vi "Data_get.vi"() -> ()   [LabVIEW 2009]
uses:
  <vilib>/Analysis/2dsp.llb/Real FFT.vi
  <vilib>/Analysis/NI_AALPro.lvlib
panel:
  in  "Chirp up to (GHz)":dbl
  in  "PauseB":bool caption="Pause"
  in  "Substr":bool
  out "tdsavges#":i32 caption="tds averaged:"
  in  "Auto":bool caption="Autosave"
  in  "FFT every#":u32=1 min=1 max=1000 step=1
  in  "#steps":u32=1 min=1 step=1
  in  "f step (MHz)":dbl=0.0003 min=0.00025 max=67.0 step=1e-06 format="%#.12f"
  in  "ps/point":T1(ring)
  in  "ns/div":T2(ring)
  out "Current sweep":u32=1 min=1 max=1000 step=1
  in  "Ext":string="ccd"
  out "f cur. (MHz)":string
  in  "Name":string="trace"
  in  "Folder":path
  in  "#Sweeps":u32=1 min=1 max=1000 step=1
  in  "Ampl. (dBm)":dbl min=-135.0 max=30.0 step=0.5 format="%#_8g"
  in  "f start (MHz)":dbl=0.0003 min=0.00025 max=67.0 step=1e-06 format="%#.12f"
  in  "Start":bool
  in  "Quit":bool
  in  "E8257D VISA Port":refnum<visa-resource-name>="GPIB0::1::INSTR"
  out "read time (ms)":u32
  out "#points":u32
  out "Busy":bool
  in  "Repetition rate (Hz)":ext=2.5
  in  "Chirp start (MHz)":ext=2.5
  in  "Filter up to (MHz)":ext=2.5
  in  "Amount of averagings":u32=10 min=1 step=1
  out "Data":dbl[](array[numeric])
  out "XY Graph 5":cluster{ext[], dbl[]}(graph)
  out "FFT (Im)":dbl[](array[numeric])
  out "FFT (Re)":dbl[](array[numeric])
  out "Final array":ext[][](array[numeric])
  out "size(s)":i32
  out "Oscilloscope Data":dbl[](array[numeric])
  in  "Channel Number":u16=1
  out "Oscilloscope graph":dbl[](graph)
  in  "Stop":bool
  in  "TDS VISA Port":refnum<visa-resource-name>="GPIB0::1::INSTR"
  # "TDS6000"
  # "E8257D"
  # "File Storage"
  # "Control"
  # "Spectrum data"
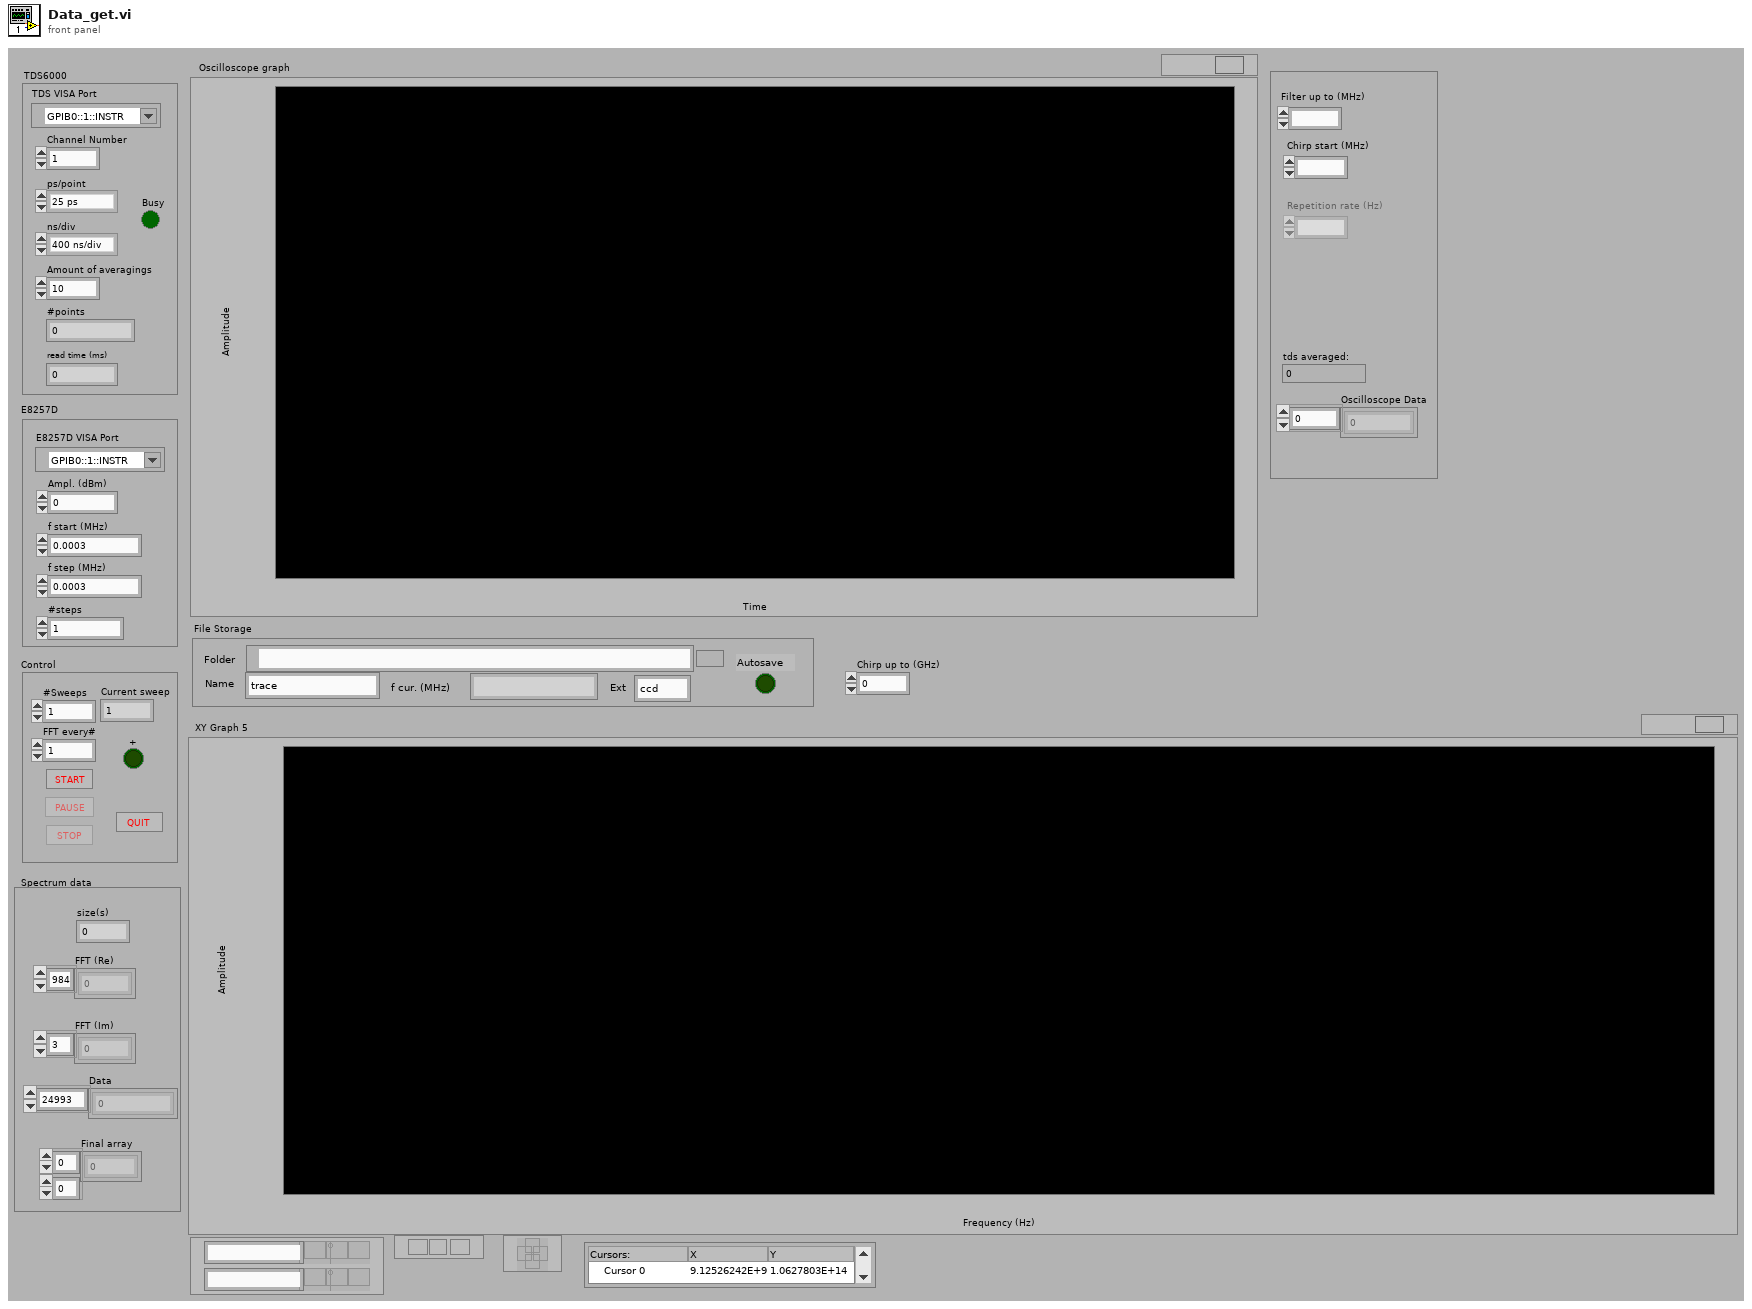
[diagram p1: front panel]
types:
  T1 = enum16{"25 ps", "50 ps", "100 ps", "200 ps", "400 ps", "800 ps", "2 ns"}
  T2 = enum16{"400 ns/div", "1 us/div", "2 us/div", "4 us/div", "10 us/div", "20 us/div"}
  T3 = enum8{"Enabled", "Disabled", "Disabled and Grayed Out"}
  T4 = enum16{"open", "replace", "create", "open or create", "replace or create", "replace or create with confirmation"}
  T5 = cluster{"Folder":path, "Name":string, "Ext":string}
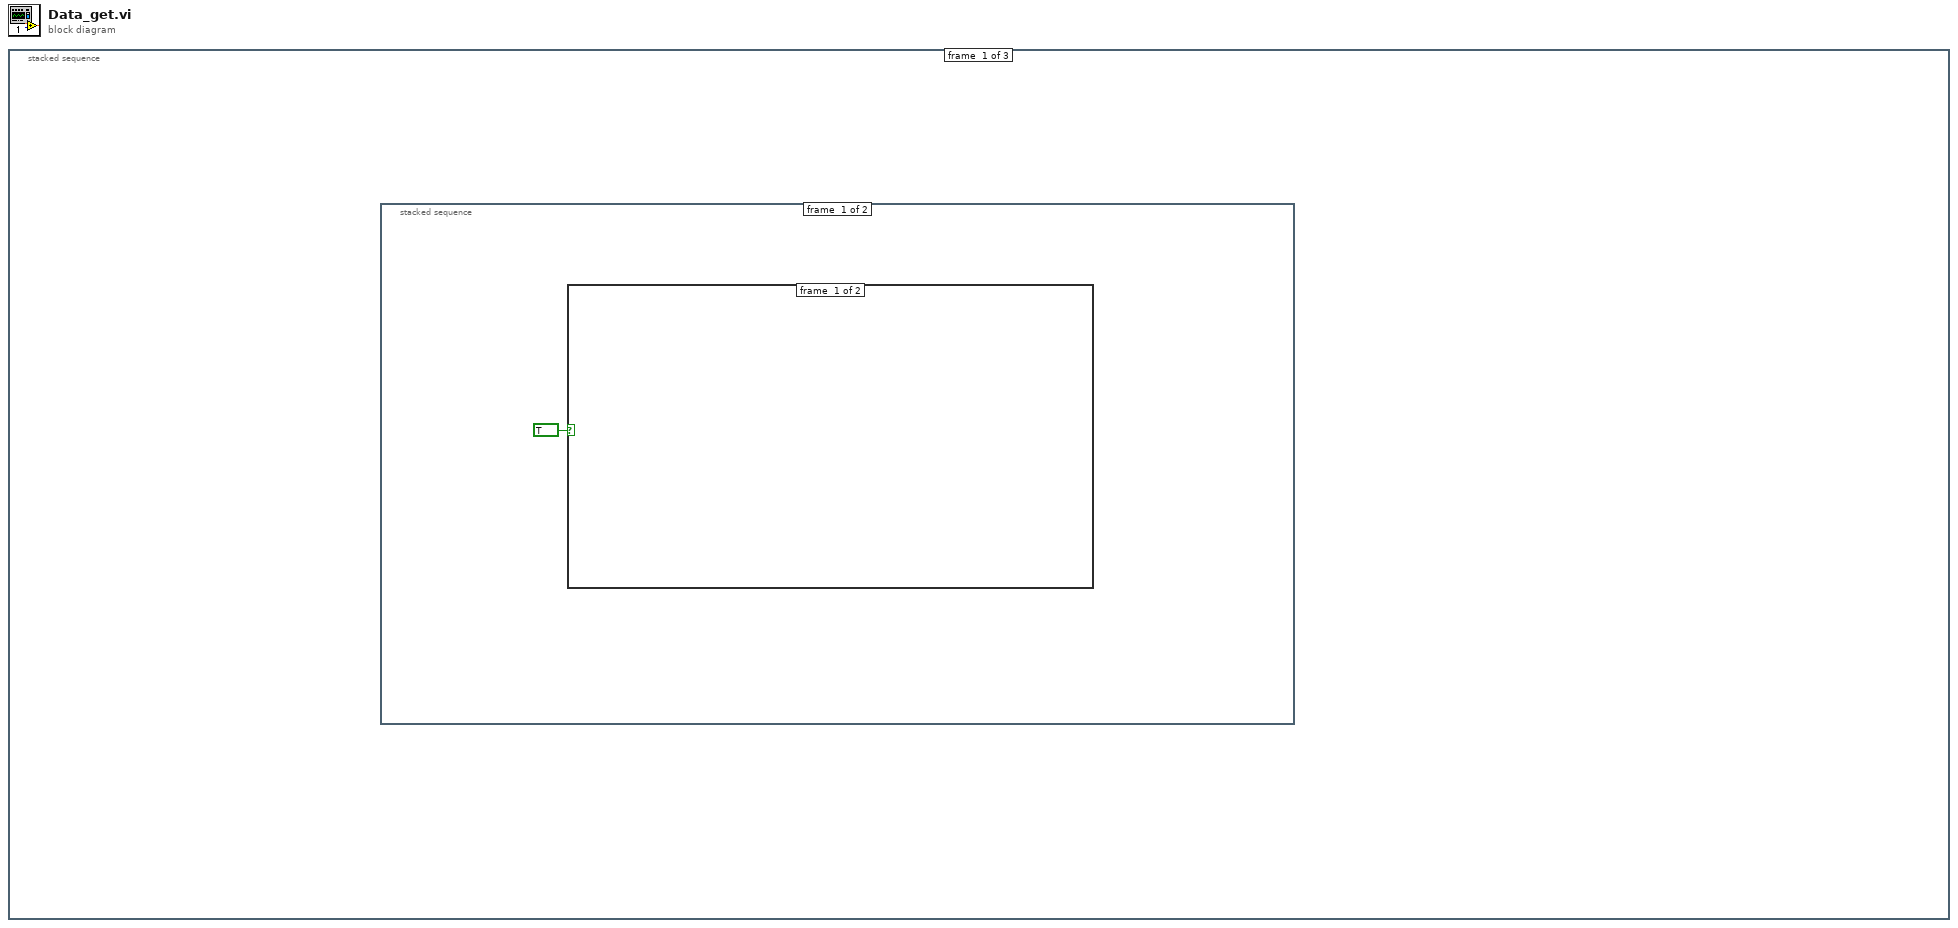
[diagram p0: block diagram]
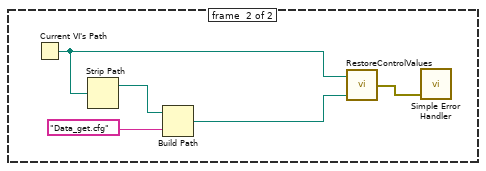
[diagram p2: hidden frame]
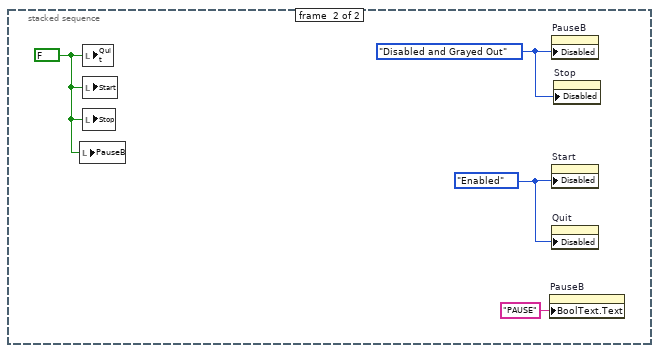
[diagram p3: hidden frame]
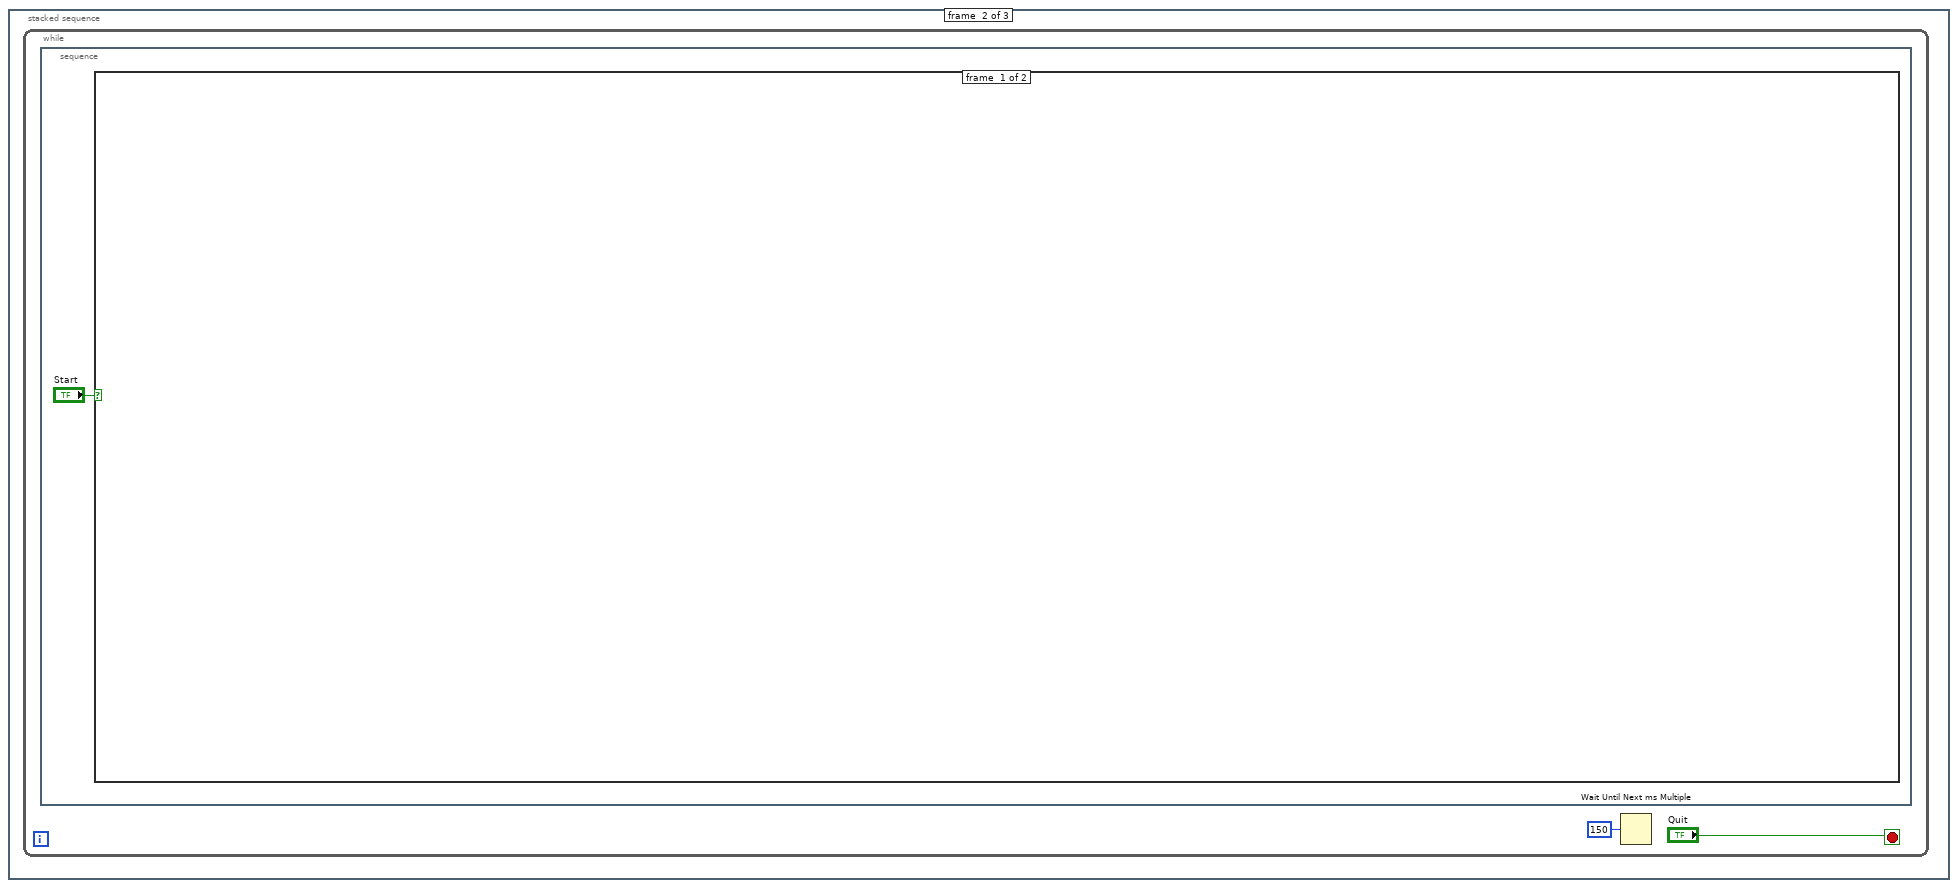
[diagram p4: hidden frame]
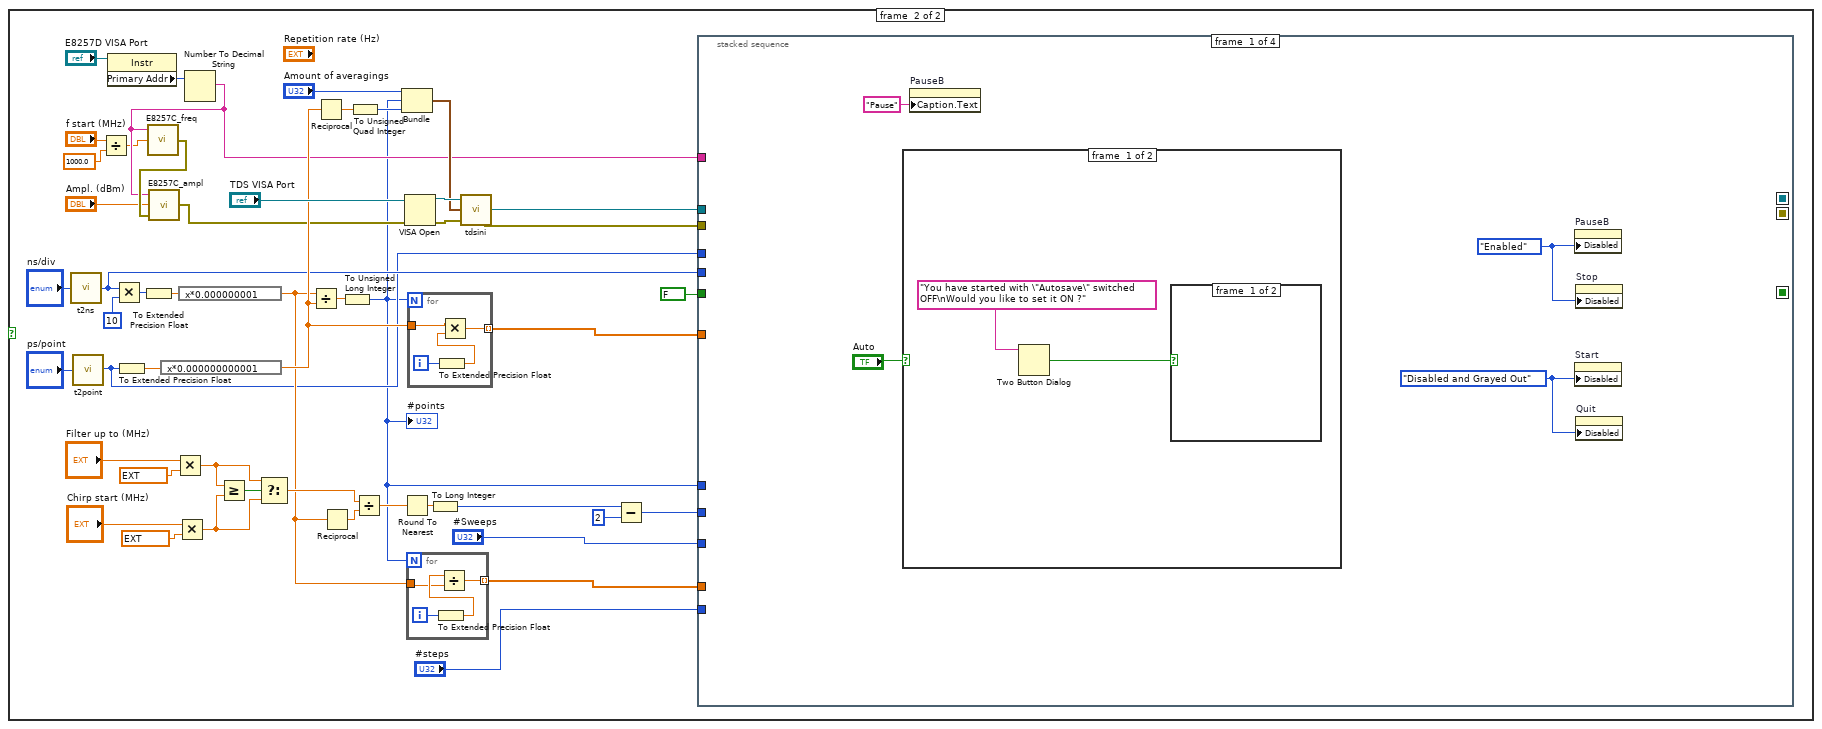
[diagram p5: hidden frame]
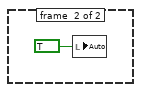
[diagram p6: hidden frame]
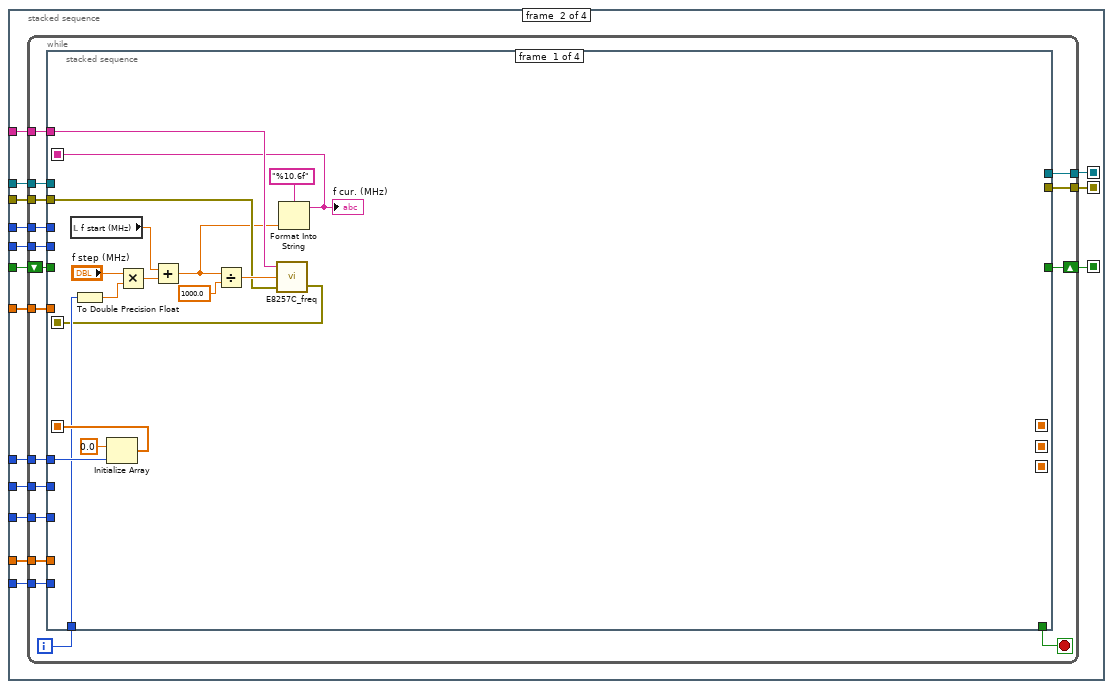
[diagram p8: hidden frame]
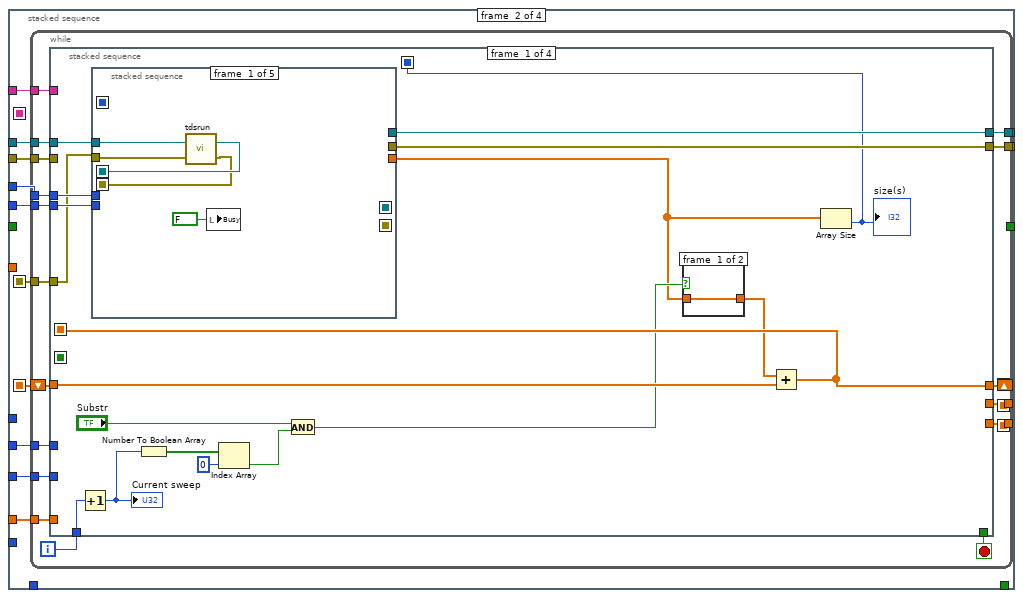
[diagram p9: hidden frame]
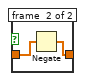
[diagram p10: hidden frame]
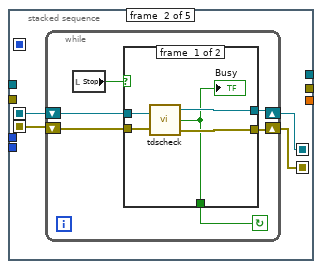
[diagram p11: hidden frame]
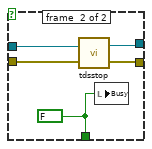
[diagram p12: hidden frame]
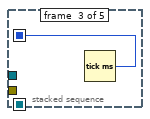
[diagram p13: hidden frame]
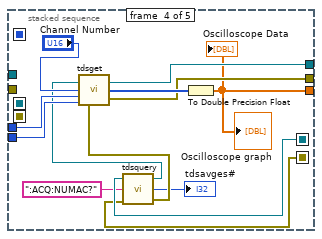
[diagram p14: hidden frame]
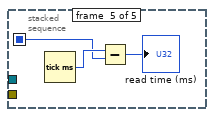
[diagram p15: hidden frame]
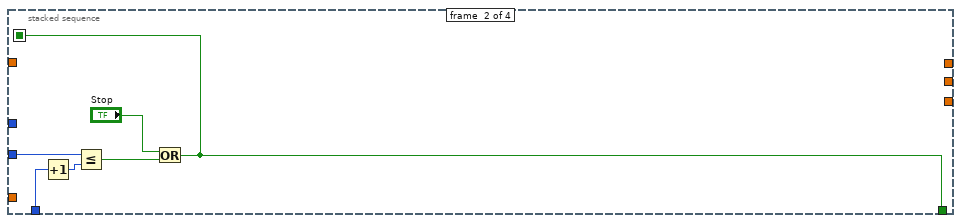
[diagram p16: hidden frame]
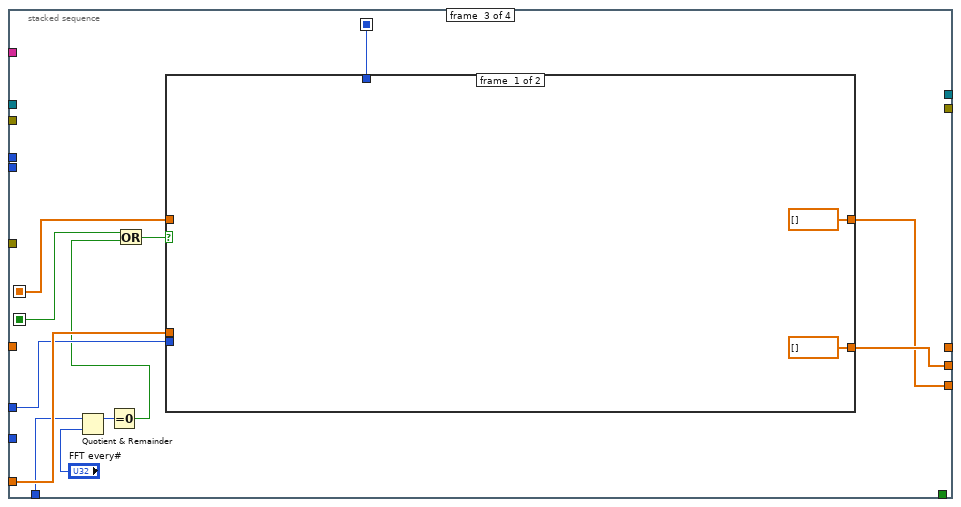
[diagram p17: hidden frame]
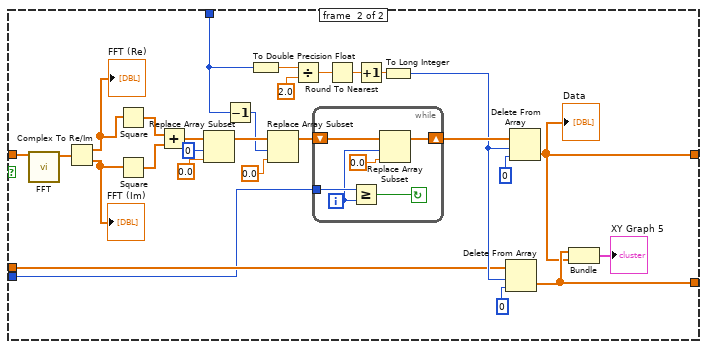
[diagram p18: hidden frame]
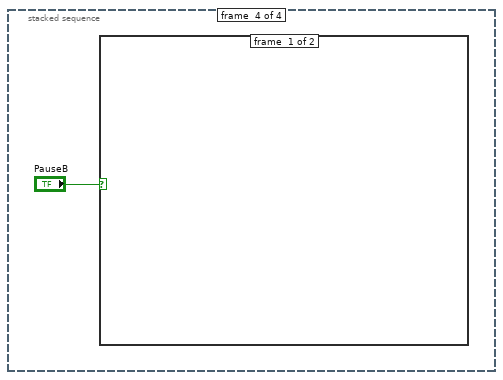
[diagram p19: hidden frame]
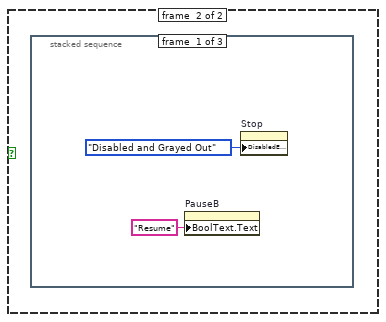
[diagram p20: hidden frame]
diagram:
  n1 = stacked-sequence {
    frame #0 {
      n2 = stacked-sequence {
        frame #0 {
          n3 = case shown="True" TRUE {
            frame #0 {
            }
            frame #1 {
              n4 = Current VI's Path() -> (path=w2:path)
              n5 = Strip Path(path=w2) -> (stripped path=w3:path)  [unwired: 1 out]
              n6 = Build Path(base path=w3, name or relative path="Data_get.cfg") -> (appended path=w5:path)
              n7 = call "RestoreControlValues.vi"("file path"=w5, "vi path"=w2) -> ("error out"=w4:errorcluster)
              n8 = call <vilib>:"Simple Error Handler.vi"("error in (no error)"=w4) -> ()  [unwired: 4 in, 5 out]
            }
          }
        }
        frame #1 {
          w9 = T3."Disabled and Grayed Out" ("Disabled")
          w7 = T3."Enabled" ("Disabled")
          w10 = FALSE ("Quit")
          n9 = local write "PauseB"(w10) -> ()
          n10 = local write "Quit"(w10) -> ()
          n11 = local write "Start"(w10) -> ()
          n12 = local write "Stop"(w10) -> ()
          n13 = property on="PauseB" class="Bool (strict)"("BoolText.Text"="PAUSE" ("Boolean Text.Text")) -> ()  [unwired: 2 in, 2 out]
          n14 = property on="PauseB" class="Bool (strict)"("Disabled"=w9) -> ()  [unwired: 2 in, 2 out]
          n15 = property on="Start" class="Bool (strict)"("Disabled"=w7) -> ()  [unwired: 2 in, 2 out]
          n16 = property on="Quit" class="Bool (strict)"("Disabled"=w7) -> ()  [unwired: 2 in, 2 out]
          n17 = property on="Stop" class="Bool (strict)"("Disabled"=w9) -> ()  [unwired: 2 in, 2 out]
        }
      }
    }
    frame #1 {
      n18 = while {
        stop <- "Quit" stop-if-true
        n19 = stacked-sequence {
          frame #0 {
            n20 = case shown="True" "Start" {
              frame #0 {
              }
              frame #1 {
                n21 = call "t2ns.vi"("t/div"="ns/div") -> ("ns/div"=w23:u32)
                n22 = call "t2point.vi"("t/point"="ps/point") -> ("ps/point"=w21:u32)
                n23 = Divide(x="f start (MHz)", y=1000.0) -> (x/y=w26:dbl)
                n24 = property class="Instr"(reference="E8257D VISA Port") -> ("Primary Addr"=w33:u16)  [unwired: 1 in, 2 out]
                n25 = Multiply(x=w23, y=u32 10) -> (x*y=w56:u32)
                n26 = To Extended Precision Float(1:w21) -> (0:w53:ext)
                n27 = To Extended Precision Float(1:w56) -> (0:w54:ext)
                n28 = expression code="x*0.000000000001"(w53) -> (w39:ext)
                n29 = Multiply(x="Filter up to (MHz)", y=ext 1000000.0) -> (x*y=w45:ext)
                n30 = Multiply(x="Chirp start (MHz)", y=ext 1000000.0) -> (x*y=w42:ext)
                n31 = expression code="x*0.000000001"(w54) -> (w35:ext)
                n32 = Number To Decimal String(number=w33) -> (decimal integer string=w30:string)  [unwired: 1 in]
                n33 = call "E8257C_freq.vi"("Frequency GHz"=w26, "GPIB address"=w30) -> ("error out"=w31:errorcluster)  [unwired: 1 in]
                n34 = call "E8257C_ampl.vi"("error in"=w31, "Amplitude dBm"="Ampl. (dBm)", "GPIB address"=w30) -> ("error out"=w29:errorcluster)
                n35 = Greater Or Equal?(x=w45, y=w42) -> (x >= y?=w52:bool)
                n36 = Select(t=w45, s=w52, f=w42) -> (s? t:f=w50:ext)
                n37 = Divide(x=w35, y=w39) -> (x/y=w55:ext)
                n38 = Reciprocal(x=w39) -> (1/x=w37:ext)
                n39 = Reciprocal(x=w35) -> (1/x=w51:ext)
                n40 = To Unsigned Long Integer(number=w55) -> (unsigned 32bit integer=w19:u32)
                "#points" <- w19
                n41 = To Unsigned Quad Integer(1:w37) -> (0:w38:u64)
                n42 = Divide(x=w50, y=w51) -> (x/y=w49:ext)
                n43 = Bundle("Amount of averagings"="Amount of averagings", w19, w38) -> (w40:cluster{"Amount of averagings ":u32, u32, u64})  [unwired: 1 in]
                n44 = Round To Nearest(number=w49) -> (nearest integer value=w48:ext)
                n45 = VISA Open(error in (no error)=w29, VISA resource name="TDS VISA Port") -> (VISA resource name=w59:refnum<visa-resource-name>, error out=w60:errorcluster)  [unwired: 3 in]
                n46 = for {
                  N: w19 -> [_]
                  tunnel: w35 -> [w468]
                  tunnel: [w470] -> w36 mode=indexing
                  i -> [w471]
                  n47 = To Extended Precision Float(1:w471) -> (0:w469:ext)
                  n48 = Divide(x=w469, y=w468) -> (x/y=w470:ext)
                }
                n49 = for {
                  N: w19 -> [_]
                  tunnel: w39 -> [w473]
                  tunnel: [w472] -> w24 mode=indexing
                  i -> [w475]
                  n50 = To Extended Precision Float(1:w475) -> (0:w474:ext)
                  n51 = Multiply(x=w473, y=w474) -> (x*y=w472:ext)
                }
                n52 = To Long Integer(number=w48) -> (32bit integer=w16:i32)
                n53 = call "tdsini.vi"("Error In (No Error)"=w60, "Acq_par"=w40, "VISA Port In"=w59) -> ("Error Out"=w61:errorcluster, "VISA Port Out"=w62:refnum<visa-resource-name>)
                n54 = Subtract(x=w16, y=2) -> (x-y=w14:i32)
                n55 = stacked-sequence {
                  seq-local: [_ w76 _ _] -> [_ _ w429 _]
                  seq-local: [_ w75 _ _] -> [_ _ w428 _]
                  seq-local: [_ w70 _ _] -> [_ _ _ w430]
                  tunnel: w62 -> [_ w84 _ _]
                  tunnel: w61 -> [_ w83 _ _]
                  tunnel: w21 -> [_ w82 _ _]
                  tunnel: w23 -> [_ w81 _ _]
                  tunnel: w14 -> [_ w80 _ _]
                  tunnel: w36 -> [_ w79 _ _]
                  tunnel: w30 -> [_ w78 w426 _]
                  tunnel: "#Sweeps" -> [_ w77 _ _]
                  tunnel: w24 -> [_ w72 _ _]
                  tunnel: w19 -> [_ w74 _ _]
                  tunnel: "#steps" -> [_ w73 _ _]
                  tunnel: FALSE -> [_ w71 _ _]
                  frame #0 {
                    w64 = T3."Enabled" ("Disabled")
                    w63 = T3."Disabled and Grayed Out" ("Disabled")
                    n56 = case shown="False" "Auto" {
                      frame #0 {
                        n57 = Two Button Dialog(message="You have started with \"Autosave\" switched OFF\nWould you like to set it ON ?") -> (T button?=w67:bool)  [unwired: 2 in]
                        n58 = case shown="True" w67 {
                          frame #0 {
                          }
                          frame #1 {
                            n59 = local write "Auto"(TRUE) -> ()
                          }
                        }
                      }
                      frame #1 {
                      }
                    }
                    n60 = property on="PauseB" class="Bool (strict)"("Caption.Text"="Pause") -> ()  [unwired: 2 in, 2 out]
                    n61 = property on="PauseB" class="Bool (strict)"("Disabled"=w64) -> ()  [unwired: 2 in, 2 out]
                    n62 = property on="Start" class="Bool (strict)"("Disabled"=w63) -> ()  [unwired: 2 in, 2 out]
                    n63 = property on="Stop" class="Bool (strict)"("Disabled"=w64) -> ()  [unwired: 2 in, 2 out]
                    n64 = property on="Quit" class="Bool (strict)"("Disabled"=w63) -> ()  [unwired: 2 in, 2 out]
                  }
                  frame #1 {
                    n65 = while {
                      tunnel: w84 -> [w101]
                      tunnel: w83 -> [w100]
                      tunnel: w82 -> [w99]
                      tunnel: w81 -> [w98]
                      tunnel: w80 -> [w97]
                      tunnel: w79 -> [w96]
                      tunnel: w78 -> [w95]
                      tunnel: w77 -> [w94]
                      tunnel: [w93] -> w76
                      tunnel: [w92] -> w75
                      tunnel: w74 -> [w91]
                      tunnel: w73 -> [w89]
                      tunnel: w72 -> [w87]
                      shift-right: [w85] -> w70
                      shift-left: w71 -> [w86]
                      i -> [w90]
                      stop <- w88 stop-if-true
                      n66 = stacked-sequence {
                        seq-local: [w116 _ _ _] -> [_ w122 _ _]
                        seq-local: [w105 _ _ _] -> [_ w121 _ _]
                        seq-local: [_ w120 _ _] -> [_ _ w280 _]
                        seq-local: [_ w119 _ _] -> [_ _ w279 _]
                        seq-local: [_ w118 _ _] -> [_ _ w278 _]
                        seq-local: [w102 _ _ _] -> [_ _ w277 _]
                        tunnel: w101 -> [_ w132 _ _]
                        tunnel: w100 -> [w106 w131 _ _]
                        tunnel: w99 -> [_ w130 _ _]
                        tunnel: w98 -> [_ w129 _ _]
                        tunnel: w97 -> [_ w128 _ _]
                        tunnel: w96 -> [_ w127 _ _]
                        tunnel: w95 -> [w107 w126 _ _]
                        tunnel: w94 -> [_ w125 _ _]
                        tunnel: [_ w124 _ _] -> w93
                        tunnel: [_ w123 _ _] -> w92
                        tunnel: w91 -> [w115 _ _ _]
                        tunnel: w90 -> [w110 _ _ w420]
                        tunnel: w89 -> [_ _ _ w419]
                        tunnel: [_ _ _ w418] -> w88
                        tunnel: w87 -> [_ _ w281 _]
                        tunnel: w86 -> [_ _ w275 _]
                        tunnel: [_ _ w274 _] -> w85
                        frame #0 {
                          n67 = local read "f start (MHz)"() -> (w108:dbl)
                          n68 = To Double Precision Float(number=w110) -> (double precision float=w111:dbl)
                          n69 = Initialize Array(0.0 ("element"), w115) -> (w116:dbl[])
                          n70 = Multiply(x="f step (MHz)", y=w111) -> (x*y=w109:dbl)
                          n71 = Add(x=w108, y=w109) -> (x+y=w104:dbl)
                          n72 = Divide(x=w104, y=1000.0) -> (x/y=w114:dbl)
                          n73 = call "E8257C_freq.vi"("error in"=w106, "Frequency GHz"=w114, "GPIB address"=w107) -> ("error out"=w105:errorcluster)
                          n74 = Format Into String(format string="%10.6f", w104) -> (resulting string=w102:string)  [unwired: 2 in, 1 out]
                          "f cur. (MHz)" <- w102
                        }
                        frame #1 {
                          n75 = while {
                            tunnel: [w146] -> w123
                            tunnel: [w147] -> w124
                            tunnel: w131 -> [w148]
                            tunnel: w132 -> [w149]
                            tunnel: w130 -> [w145]
                            tunnel: w129 -> [w144]
                            tunnel: w127 -> [w142]
                            tunnel: w128 -> [w143]
                            tunnel: w126 -> [w139]
                            tunnel: w125 -> [w138]
                            shift-right: [w136] -> w120
                            shift-left: w122 -> [w137]
                            tunnel: [w135] -> w119
                            tunnel: w121 -> [w134]
                            tunnel: [w133] -> w118
                            i -> [w141]
                            stop <- w140 stop-if-true
                            n76 = stacked-sequence {
                              seq-local: [w159 _ _ _] -> [_ _ w230 _]
                              seq-local: [w160 _ _ _] -> [_ _ w229 _]
                              seq-local: [_ w213 _ _] -> [_ _ w220 _]
                              tunnel: w149 -> [w167 _ _ _]
                              tunnel: w148 -> [_ _ _ _]
                              tunnel: [w166 _ _ _] -> w147
                              tunnel: [w165 _ _ _] -> w146
                              tunnel: w145 -> [w164 _ _ _]
                              tunnel: w144 -> [w163 _ _ _]
                              tunnel: w143 -> [_ _ w227 _]
                              tunnel: w142 -> [_ _ w228 _]
                              tunnel: w141 -> [w158 w218 w224 _]
                              tunnel: [_ w213 _ _] -> w140
                              tunnel: w139 -> [_ _ _ _]
                              tunnel: w138 -> [_ w215 _ _]
                              tunnel: w137 -> [w162 _ _ _]
                              tunnel: [w160 _ _ _] -> w136
                              tunnel: [_ _ w226 _] -> w135
                              tunnel: w134 -> [w161 _ _ _]
                              tunnel: [_ _ w225 _] -> w133
                              frame #0 {
                                n77 = Increment(x=w158) -> (x+1=w150:i32)
                                "Current sweep" <- w150
                                n78 = stacked-sequence {
                                seq-local: [w173 _ _ _ _] -> [_ w179 _ _ _]
                                seq-local: [w172 _ _ _ _] -> [_ w178 _ _ _]
                                seq-local: [_ w176 _ _ _] -> [_ _ _ w201 _]
                                seq-local: [_ w177 _ _ _] -> [_ _ _ w202 _]
                                seq-local: [_ _ w196 _ _] -> [_ _ _ _ w211]
                                tunnel: w167 -> [w174 _ _ _ _]
                                tunnel: w161 -> [w175 _ _ _ _]
                                tunnel: [_ _ _ w208 _] -> w166
                                tunnel: [_ _ _ w207 _] -> w165
                                tunnel: w164 -> [_ _ _ w205 _]
                                tunnel: w163 -> [_ _ _ w204 _]
                                tunnel: [_ _ _ w203 _] -> w153
                                frame #0 {
                                n79 = call "tdsrun.vi"("Error In (No Error)"=w175, "VISA Port In"=w174) -> ("Error Out"=w172:errorcluster, "VISA Port Out"=w173:refnum<visa-resource-name>)
                                n80 = local write "Busy"(FALSE ("Busy")) -> ()
                                }
                                frame #1 {
                                n81 = while {
                                shift-right: [w183] -> w177
                                shift-left: w179 -> [w184]
                                shift-right: [w182] -> w176
                                shift-left: w178 -> [w185]
                                stop <- w181 continue-if-true
                                n82 = local read "Stop"() -> (w180:bool)
                                n83 = case shown="True" w180 {
                                tunnel: w185 -> [w190 w194]
                                tunnel: w184 -> [w189 w195]
                                tunnel: [w188 w192] -> w183
                                tunnel: [w187 w193] -> w182
                                tunnel: [w186 w191] -> w181
                                frame #0 {
                                n84 = call "tdscheck.vi"("VISA Port In"=w189, "Error In (No Error)"=w190) -> ("VISA Port Out"=w188:refnum<visa-resource-name>, "busy"=w186:bool, "Error Out"=w187:errorcluster)
                                "Busy" <- w186
                                }
                                frame #1 {
                                w191 = FALSE ("busy")
                                n85 = call "tdsstop.vi"("Error In (No Error)"=w194, "VISA Port In"=w195) -> ("Error Out"=w193:errorcluster, "VISA Port Out"=w192:refnum<visa-resource-name>)
                                n86 = local write "Busy"(w191) -> ()
                                }
                                }
                                }
                                }
                                frame #2 {
                                n87 = Tick Count (ms)() -> (millisecond timer value=w196:u32)
                                }
                                frame #3 {
                                n88 = call "tdsquery.vi"("Error In (No Error)"=w201, "String to TDS"=":ACQ:NUMAC?", "VISA Port In"=w202) -> ("Error Out"=w198:errorcluster, "number"=→"tdsavges#":i32, "VISA Port Out"=w199:refnum<visa-resource-name>)
                                n89 = call "tdsget.vi"("VISA Port In"=w199, "Channel Number"="Channel Number", "ps/point"=w205, "ns/div"=w204, "Error In (No Error)"=w198) -> ("VISA Port Out"=w208:refnum<visa-resource-name>, "TDS Data"=w209:u16[], "Error Out"=w207:errorcluster)  [unwired: 8 in]
                                n90 = To Double Precision Float(number=w209) -> (double precision float=w203:dbl[])
                                "Oscilloscope graph" <- w203
                                "Oscilloscope Data" <- w203
                                }
                                frame #4 {
                                n91 = Tick Count (ms)() -> (millisecond timer value=w212:u32)
                                n92 = Subtract(x=w212, y=w211) -> (x-y=→"read time (ms)":u32)
                                }
                                }
                                n93 = Number To Boolean Array(number=w150) -> (Boolean array=w157:bool[])
                                n94 = Index Array(array=w157, index=0) -> (element=w155:bool)
                                n95 = And(x="Substr", y=w155) -> (x .and. y?=w154:bool)
                                n96 = case shown="True" w154 {
                                tunnel: w153 -> [w168 w170]
                                tunnel: [w168 w169] -> w152
                                frame #0 {
                                }
                                frame #1 {
                                n97 = Negate(x=w170) -> (-x=w169:dbl[])
                                }
                                }
                                n98 = Add(x=w152, y=w162) -> (x+y=w160:dbl[])
                                n99 = Array Size(array=w153) -> (size(s)=w159:i32)
                                "size(s)" <- w159
                              }
                              frame #1 {
                                n100 = Increment(x=w218) -> (x+1=w214:i32)
                                n101 = Less Or Equal?(x=w215, y=w214) -> (x <= y?=w217:bool)
                                n102 = Or(x="Stop", y=w217) -> (x .or. y?=w213:bool)
                              }
                              frame #2 {
                                n103 = Quotient & Remainder(x=w224, y="FFT every#") -> (x-y*floor(x/y)=w222:u32)  [unwired: 1 out]
                                n104 = Equal To 0?(x=w222) -> (x = 0?=w219:bool)
                                n105 = Or(x=w220, y=w219) -> (x .or. y?=w221:bool)
                                n106 = case shown="True" w221 {
                                tunnel: w230 -> [_ w238]
                                tunnel: w229 -> [_ w237]
                                tunnel: w228 -> [_ w236]
                                tunnel: w227 -> [_ w235]
                                tunnel: [ext[] [] w234] -> w226
                                tunnel: [dbl[] [] w233] -> w225
                                frame #0 {
                                }
                                frame #1 {
                                n107 = call-poly <vilib>:"FFT.vi"("X"=w237) -> ("FFT {X}"=w260:cdb[])  [unwired: 9 in, 1 out]
                                n108 = Complex To Re/Im(x + iy=w260) -> (x=w259:dbl[], y=w258:dbl[])
                                "FFT (Re)" <- w259
                                "FFT (Im)" <- w258
                                n109 = Square(x=w259) -> (x^2=w257:dbl[])
                                n110 = Square(x=w258) -> (x^2=w256:dbl[])
                                n111 = Add(x=w257, y=w256) -> (x+y=w252:dbl[])
                                n112 = Replace Array Subset(array=w252, new element=0.0 ("new element/subarray"), index=0) -> (w251:dbl[])
                                n113 = Decrement(x=w238) -> (x-1=w250:i32)
                                n114 = To Double Precision Float(number=w238) -> (double precision float=w246:dbl)
                                n115 = Replace Array Subset(array=w251, new element=0.0 ("new element/subarray"), index=w250) -> (w248:dbl[])
                                n116 = Divide(x=w246, y=2.0) -> (x/y=w244:dbl)
                                n117 = while {
                                tunnel: w235 -> [w265]
                                shift-right: [w263] -> w247
                                shift-left: w248 -> [w264]
                                i -> [w262]
                                stop <- w266 continue-if-true
                                n118 = Greater Or Equal?(x=w265, y=w262) -> (x >= y?=w266:bool)
                                n119 = Replace Array Subset(array=w264, new element=0.0 ("new element/subarray"), index=w262) -> (w263:dbl[])
                                }
                                n120 = Round To Nearest(number=w244) -> (nearest integer value=w243:dbl)
                                n121 = Increment(x=w243) -> (x+1=w242:dbl)
                                n122 = To Long Integer(number=w242) -> (32bit integer=w239:i32)
                                n123 = Delete From Array(array=w236, length=w239, index=0) -> (deleted portion=w234:ext[])  [unwired: 1 out]
                                n124 = Delete From Array(array=w247, length=w239, index=0) -> (deleted portion=w233:dbl[])  [unwired: 1 out]
                                "Data" <- w233
                                n125 = Bundle(w234, w233) -> (→"XY Graph 5":cluster{ext[], dbl[]})  [unwired: 1 in]
                                }
                                }
                              }
                              frame #3 {
                                n126 = case shown="True" "PauseB" {
                                frame #0 {
                                }
                                frame #1 {
                                n127 = stacked-sequence {
                                frame #0 {
                                n128 = property on="PauseB" class="Bool (strict)"("BoolText.Text"="Resume" ("Caption.Text")) -> ()  [unwired: 2 in, 2 out]
                                n129 = property on="Stop" class="Bool (strict)"("DisabledEnum"=T3."Disabled and Grayed Out" ("Disabled")) -> ()  [unwired: 2 in, 2 out]
                                }
                                frame #1 {
                                n130 = while {
                                stop <- w271 continue-if-true
                                n131 = local read "PauseB"() -> (w271:bool)
                                n132 = Wait Until Next ms Multiple(millisecond multiple=u32 150) -> ()  [unwired: 1 out]
                                }
                                }
                                frame #2 {
                                n133 = property on="PauseB" class="Bool (strict)"("BoolText.Text"="Pause" ("Caption.Text")) -> ()  [unwired: 2 in, 2 out]
                                n134 = property on="Stop" class="Bool (strict)"("DisabledEnum"=T3."Enabled" ("Disabled")) -> ()  [unwired: 2 in, 2 out]
                                }
                                }
                                }
                                }
                              }
                            }
                          }
                        }
                        frame #2 {
                          n135 = local read "Auto"() -> (w276:bool)
                          n136 = case shown="True" w276 {
                            tunnel: w281 -> [_ w289]
                            tunnel: w280 -> [_ w288]
                            tunnel: w279 -> [_ w287]
                            tunnel: w278 -> [_ w286]
                            tunnel: w277 -> [_ w285]
                            tunnel: w275 -> [_ w284]
                            tunnel: [FALSE w283] -> w274
                            frame #0 {
                            }
                            frame #1 {
                              n137 = stacked-sequence {
                                seq-local: [w290 _ _ _] -> [_ w315 _ _]
                                seq-local: [_ _ w370 _] -> [_ _ _ w410]
                                seq-local: [_ w302 _ _] -> [_ _ _ w401]
                                tunnel: w289 -> [_ w317 _ _]
                                tunnel: w288 -> [_ w304 _ _]
                                tunnel: w287 -> [_ _ _ w413]
                                tunnel: w286 -> [_ _ _ w412]
                                tunnel: w285 -> [w292 w303 w372 _]
                                tunnel: w284 -> [_ w307 _ _]
                                tunnel: [_ w302 _ _] -> w283
                                frame #0 {
                                n138 = Path To String(path="Folder") -> (string=w300:string)
                                n139 = Concatenate Strings(w300, "\\\\" ("string"), "Name", "_") -> (w291:string)
                                n140 = Concatenate Strings(w291, "td", w292, ".", "Ext") -> (w290:string)
                                }
                                frame #1 {
                                n141 = String To Path(string=w315) -> (path=w306:path)
                                n142 = case shown="False" w307 {
                                tunnel: w315 -> [w321 _]
                                tunnel: [w326 w368] -> w302
                                tunnel: [w324 T4."replace or create" ("operation (0:open)")] -> w309
                                tunnel: w307 -> [w325 w368]
                                tunnel: w306 -> [w323 w367]
                                tunnel: [w322 w367] -> w305
                                tunnel: w303 -> [w320 _]
                                frame #0 {
                                n143 = call "CheckFileExist.vi"("Path"=w321) -> ("Exist"=w328:bool, "Overwrite"=w327:bool)  [unwired: 1 in, 1 out]
                                n144 = case shown="True" w328 {
                                tunnel: w327 -> [_ w337]
                                tunnel: [w331 w335] -> w326
                                tunnel: w325 -> [w331 _]
                                tunnel: [T4."create" ("operation (0:open)") w336] -> w324
                                tunnel: w323 -> [w329 w334]
                                tunnel: [w329 w333] -> w322
                                tunnel: w320 -> [_ w332]
                                frame #0 {
                                }
                                frame #1 {
                                n145 = case shown="True" w337 {
                                tunnel: [w340 T4."replace or create" ("operation (0:open)")] -> w336
                                tunnel: [w341 TRUE] -> w335
                                tunnel: w334 -> [_ w364]
                                tunnel: [w338 w364] -> w333
                                tunnel: w332 -> [w339 _]
                                frame #0 {
                                n146 = stacked-sequence {
                                tunnel: [_ _ FALSE] -> w341
                                tunnel: [_ _ T4."create" ("operation (0:open)")] -> w340
                                tunnel: w339 -> [_ w353 _]
                                tunnel: [_ w350 _] -> w338
                                frame #0 {
                                n147 = local read "Folder"() -> (w349:path)
                                n148 = local read "Name"() -> (w348:string)
                                n149 = local read "Ext"() -> (w347:string)
                                n150 = Bundle("Folder"=w349, "Name"=w348, "Ext"=w347) -> (w346:T5)  [unwired: 1 in]
                                n151 = call "ChangeFileName.vi"("input par"=w346) -> ("output par"=w345:T5)  [unwired: 1 out]
                                n152 = Unbundle(w345) -> ("Folder"=w344:path, "Name"=w343:string, "Ext"=w342:string)
                                n153 = local write "Folder"(w344) -> ()
                                n154 = local write "Name"(w343) -> ()
                                n155 = local write "Ext"(w342) -> ()
                                }
                                frame #1 {
                                n156 = local read "Folder"() -> (w358:path)
                                n157 = local read "Name"() -> (w357:string)
                                n158 = local read "Ext"() -> (w352:string)
                                n159 = Path To String(path=w358) -> (string=w361:string)
                                n160 = Concatenate Strings(w361, "\\\\" ("string"), w357, "_") -> (w354:string)
                                n161 = Concatenate Strings(w354, "td", w353, ".", w352) -> (w351:string)
                                n162 = String To Path(string=w351) -> (path=w350:path)
                                }
                                frame #2 {
                                }
                                }
                                }
                                frame #1 {
                                }
                                }
                                }
                                }
                                }
                                frame #1 {
                                }
                                }
                                n163 = Build Array(w317, w304) -> (w319:ext[][])
                                n164 = Transpose 2D Array(2D array=w319) -> (transposed array=w316:ext[][])
                                n165 = Array To Spreadsheet String(array=w316, 3:"%e") -> (spreadsheet string=w308:string)  [unwired: 1 in]
                                n166 = Open/Create/Replace File(file path (use dialog)=w305, operation (0:open)=w309, access (0:read/write)=enum16{"read/write", "read-only", "write-only"}."write-only") -> (refnum out=w311:refnum<file>, error out=w314:errorcluster)  [unwired: 3 in, 1 out]
                                n167 = Write to Text File(file (use dialog)=w311, text=w308, error in=w314) -> (refnum out=w312:refnum<file>, error out=w313:errorcluster)  [unwired: 1 in, 1 out]
                                n168 = Close File(refnum=w312, error in=w313) -> (error out=w301:errorcluster)  [unwired: 1 out]
                                n169 = call <vilib>:"Simple Error Handler.vi"("error in (no error)"=w301) -> ()  [unwired: 4 in, 5 out]
                                }
                                frame #2 {
                                n170 = local read "Folder"() -> (w374:path)
                                n171 = local read "Name"() -> (w373:string)
                                n172 = local read "Ext"() -> (w371:string)
                                n173 = Path To String(path=w374) -> (string=w380:string)
                                n174 = Concatenate Strings(w380, "\\\\" ("string"), w373, "_") -> (w375:string)
                                n175 = Concatenate Strings(w375, "sd", w372, ".", w371) -> (w370:string)
                                }
                                frame #3 {
                                n176 = Multiply(x="Chirp up to (GHz)", y=1000000000.0) -> (x*y=w382:dbl)
                                n177 = To Extended Precision Float(1:w382) -> (0:w381:ext)
                                n178 = To Extended Precision Float(1:w412) -> (0:w414:ext[])
                                n179 = Build Array(w413, w414) -> (w411:ext[][])
                                n180 = String To Path(string=w410) -> (path=w403:path)
                                n181 = case shown="True" w401 {
                                tunnel: [T4."replace or create with confirmation" ("operation (0:open)") T4."replace or create" ("operation (0:open)")] -> w402
                                frame #0 {
                                }
                                frame #1 {
                                }
                                }
                                n182 = Transpose 2D Array(2D array=w411) -> (transposed array=w384:ext[][])
                                n183 = Index Array(array=w384, index (col)=0 ("disabled index (col)")) -> (element=w394:ext[])  [unwired: 1 in]
                                n184 = Index Array(array=w394, index=1) -> (element=w396:ext)
                                n185 = Index Array(array=w394, index=0) -> (element=w395:ext)
                                n186 = Subtract(x=w396, y=w395) -> (x-y=w391:ext)
                                n187 = Divide(x=w381, y=w391) -> (x/y=w388:ext)
                                n188 = Round To Nearest(number=w388) -> (nearest integer value=w390:ext)
                                n189 = To Long Integer(number=w390) -> (32bit integer=w389:i32)
                                n190 = Increment(x=w389) -> (x+1=w385:i32)
                                n191 = Array Subset(array=w384, index (row)=0 ("index"), length (row)=w385, index (col)=0 ("index"), length (col)=w385) -> (w383:ext[][])
                                "Final array" <- w383
                                n192 = Array To Spreadsheet String(array=w383, 3:"%e") -> (spreadsheet string=w404:string)  [unwired: 1 in]
                                n193 = Open/Create/Replace File(file path (use dialog)=w403, operation (0:open)=w402, access (0:read/write)=enum16{"read/write", "read-only", "write-only"}."write-only") -> (refnum out=w406:refnum<file>, error out=w409:errorcluster)  [unwired: 3 in, 1 out]
                                n194 = Write to Text File(file (use dialog)=w406, text=w404, error in=w409) -> (refnum out=w407:refnum<file>, error out=w408:errorcluster)  [unwired: 1 in, 1 out]
                                n195 = Close File(refnum=w407, error in=w408) -> (error out=w400:errorcluster)  [unwired: 1 out]
                                n196 = call <vilib>:"Simple Error Handler.vi"("error in (no error)"=w400) -> ()  [unwired: 4 in, 5 out]
                                }
                              }
                            }
                          }
                        }
                        frame #3 {
                          n197 = Increment(x=w420) -> (x+1=w422:i32)
                          n198 = Less Or Equal?(x=w419, y=w422) -> (x <= y?=w423:bool)
                          n199 = local read "Stop"() -> (w421:bool)
                          n200 = Or(x=w421, y=w423) -> (x .or. y?=w418:bool)
                        }
                      }
                    }
                  }
                  frame #2 {
                    w425 = T3."Disabled and Grayed Out" ("Disabled")
                    w424 = T3."Enabled" ("Disabled")
                    n201 = call "E8257C_local.vi"("GPIB address"=w426) -> ("error out"=w427:errorcluster)  [unwired: 1 in]
                    n202 = call <vilib>:"Simple Error Handler.vi"("error in (no error)"=w427) -> ()  [unwired: 4 in, 5 out]
                    n203 = property on="Quit" class="Bool (strict)"("Disabled"=w424) -> ()  [unwired: 2 in, 2 out]
                    n204 = property on="PauseB" class="Bool (strict)"("Disabled"=w425) -> ()  [unwired: 2 in, 2 out]
                    n205 = property on="Stop" class="Bool (strict)"("Disabled"=w425) -> ()  [unwired: 2 in, 2 out]
                    n206 = property on="Start" class="Bool (strict)"("Disabled"=w424) -> ()  [unwired: 2 in, 2 out]
                    n207 = VISA Close(VISA resource name=w429, error in (no error)=w428) -> ()  [unwired: 1 out]
                  }
                  frame #3 {
                    n208 = local read "Auto"() -> (w431:bool)
                    n209 = case shown="True" w431 {
                      tunnel: w430 -> [_ w434]
                      frame #0 {
                      }
                      frame #1 {
                        n210 = local read "Channel Number"() -> (w464:u16)
                        n211 = local read "ps/point"() -> (w463:T1)
                        n212 = local read "ns/div"() -> (w462:T2)
                        n213 = local read "Amount of averagings"() -> (w461:u32)
                        n214 = local read "#Sweeps"() -> (w460:u32)
                        n215 = local read "Filter up to (MHz)"() -> (w459:ext)
                        n216 = local read "Chirp start (MHz)"() -> (w458:ext)
                        n217 = local read "Ampl. (dBm)"() -> (w457:dbl)
                        n218 = local read "f start (MHz)"() -> (w454:dbl)
                        n219 = local read "f step (MHz)"() -> (w453:dbl)
                        n220 = local read "#steps"() -> (w452:u32)
                        n221 = call "t2point.vi"("t/point"=w463) -> ("ps/point"=w455:u32)
                        n222 = call "t2ns.vi"("t/div"=w462) -> ("ns/div"=w456:u32)
                        n223 = local read "Folder"() -> (w448:path)
                        n224 = local read "Name"() -> (w447:string)
                        n225 = local read "Ext"() -> (w444:string)
                        n226 = Path To String(path=w448) -> (string=w451:string)
                        n227 = Format Into String(format string="Channel: %d\\nps/point: %d\\nns/div: %d\\nAmount of averagings: %d\\n#Sweeps: %d\\nFilter up to (MHz): %f\\nChirp start (MHz): %f\\nAmpl. (dBm): %f\\nf start (MHz): %f\\nf step (MHz): %f\\n#steps: %d\\n", w464, w455, w456, w461, w460, w459, w458, w457, w454, w453, w452) -> (resulting string=w435:string)  [unwired: 2 in, 1 out]
                        n228 = Concatenate Strings(w451, "\\\\" ("string"), w447, "_", "par", ".", w444) -> (w443:string)
                        n229 = case shown="False" w434 {
                          tunnel: [T4."replace or create with confirmation" ("operation (0:open)") T4."replace or create" ("operation (0:open)")] -> w433
                          frame #0 {
                          }
                          frame #1 {
                          }
                        }
                        n230 = String To Path(string=w443) -> (path=w437:path)
                        n231 = Open/Create/Replace File(file path (use dialog)=w437, operation (0:open)=w433, access (0:read/write)=enum16{"read/write", "read-only", "write-only"}."write-only") -> (refnum out=w439:refnum<file>, error out=w442:errorcluster)  [unwired: 3 in, 1 out]
                        n232 = Write to Text File(file (use dialog)=w439, text=w435, error in=w442) -> (refnum out=w440:refnum<file>, error out=w441:errorcluster)  [unwired: 1 in, 1 out]
                        n233 = Close File(refnum=w440, error in=w441) -> (error out=w438:errorcluster)  [unwired: 1 out]
                        n234 = call <vilib>:"Simple Error Handler.vi"("error in (no error)"=w438) -> ()  [unwired: 4 in, 5 out]
                      }
                    }
                    n235 = local write "Stop"(FALSE ("Stop")) -> ()
                  }
                }
              }
            }
          }
        }
        n236 = Wait Until Next ms Multiple(millisecond multiple=u32 150) -> ()  [unwired: 1 out]
      }
    }
    frame #2 {
      n237 = Current VI's Path() -> (path=w476:path)
      n238 = Strip Path(path=w476) -> (stripped path=w477:path)  [unwired: 1 out]
      n239 = Build Path(base path=w477, name or relative path="Data_get.cfg") -> (appended path=w479:path)
      n240 = call "SaveControlValues.vi"("file path"=w479, "vi path"=w476) -> ("error out"=w478:errorcluster)
      n241 = call <vilib>:"Simple Error Handler.vi"("error in (no error)"=w478) -> ()  [unwired: 4 in, 5 out]
    }
  }
